vi "iot retrieve data.vi"() -> ()   [LabVIEW 2018]
uses:
  <vilib>/httpClient/LabVIEWHTTPClient.lvlib
panel:
  out "var":dbl
  in  "stop":bool
  out "error out":errorcluster
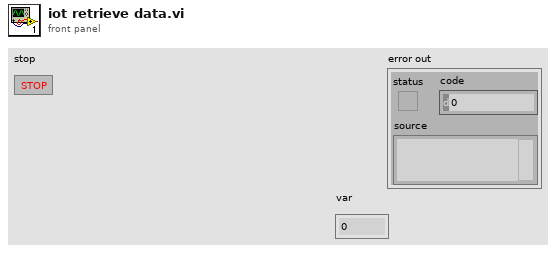
[diagram p1: front panel]
types:
  T1 = typedef "LabVIEWHTTPClient.lvlib/ClientHandle.ctl" = refnum<k1>
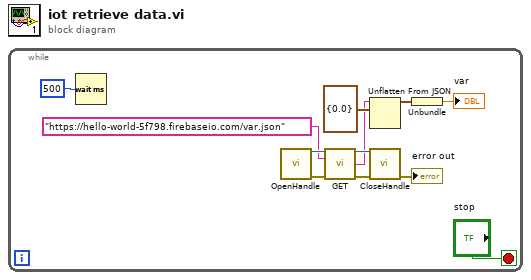
[diagram p0: block diagram]
diagram:
  n1 = while {
    stop <- "stop" stop-if-true
    n2 = Wait (ms)(milliseconds to wait=u32 500) -> ()  [unwired: 1 out]
    n3 = call <vilib>:"OpenHandle.vi"() -> ("client handle out"=w11:T1, "error out"=w9:errorcluster)  [unwired: 14 in]
    n4 = call <vilib>:"GET.vi"("client handle"=w11, "url"="https://hello-world-5f798.firebaseio.com/var.json", "error in (no error)"=w9) -> ("client handle out"=w10:T1, "body"=w5:string, "error out"=w8:errorcluster)  [unwired: 9 in, 1 out]
    n5 = Unflatten From JSON(JSON string=w5, type and defaults=cluster{"var":dbl} {"var"=0.0}) -> (value=w4:cluster{"var":dbl})  [unwired: 5 in, 1 out]
    n6 = call <vilib>:"CloseHandle.vi"("client handle"=w10, "error in (no error)"=w8) -> ("error out"=→"error out":errorcluster)  [unwired: 13 in]
    n7 = Unbundle(w4) -> ("var"=→"var":dbl)
  }
